vi "Get Result.vi"(8 "error in (no error)":errorcluster, 11 "NI-Scope Lock-in Driver in":refnum<class "NI-Scope Lock-in Driver.lvclass">) -> (0 "error out":errorcluster, 2 "Result":refnum<class "Acquired Result.lvclass">, 3 "NI-Scope Lock-in Driver out":refnum<class "NI-Scope Lock-in Driver.lvclass">)   [LabVIEW 2016, in "NI-Scope Lock-in Driver.lvclass"]
uses:
  NI-Scope Lock-in Driver.lvclass
  C:/github/NHMFL_Core/Libraries/Instruments/Pulse Driver/Pulse Driver.lvclass
  C:/github/NHMFL_Core/Libraries/Instruments/Instrument Driver/Instrument Driver.lvclass
  Instruments/Results/Acquired Result/Acquired Result.lvclass
  Instruments/Results/Start Stream Result/Start Stream Result.lvclass
  C:/github/NHMFL_Core/Libraries/Instruments/Results/Acquired Result/Acquired Result.lvclass
  NI-Scope Lock-in Driver.lvclass/NI-Scope Lock-in Driver.ctl
  Instruments/Pulse Driver/Pulse Driver.lvclass/Pulse Driver.ctl
  Instruments/Instrument Driver/Instrument Driver.lvclass/Instrument Driver.ctl
  Instruments/Results/Start Stream Result/Start Stream Result.lvclass/Start Stream Result.ctl
  Read Sine.vi
  Read Cosine.vi
  Instruments/Pulse Driver/Write Samples per read.vi
  Instruments/Instrument Driver/Read Cycle count.vi
  Instruments/Instrument Driver/Read Cycle period.vi
  Instruments/Results/Start Stream Result/Write Scaling coefficients.vi
  Instruments/Results/Start Stream Result/Write t0.vi
  Instruments/Results/Start Stream Result/Write dt.vi
  Instruments/Results/Start Stream Result/Write Configuration.vi
  Instruments/Instrument Driver/Read User configuration.vi
panel:
  out "Waveform Graph":i16[][](graph)
  out "Current read position":i32
  out "Availiable Samples":u32
  out "Sine waves read":dbl format="%.6g"
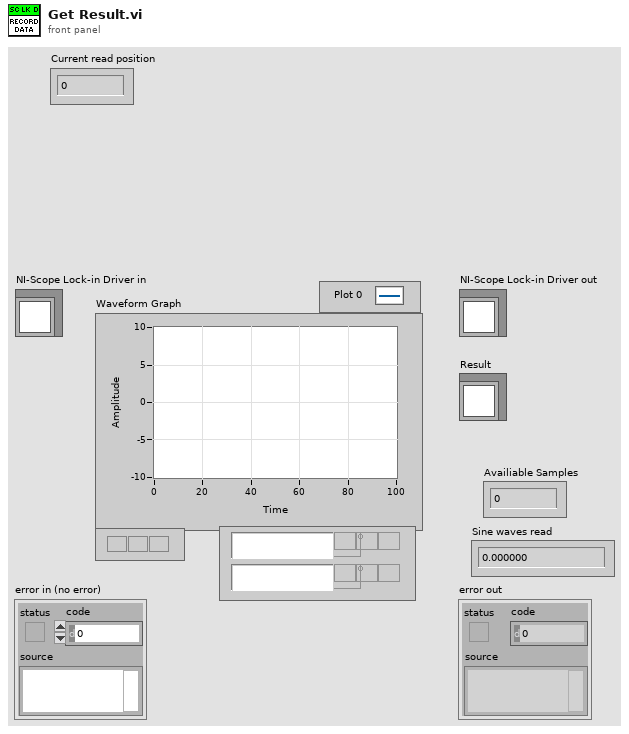
[diagram p1: front panel]
types:
  T1 = typedef "NI-Scope Lock-in Configuration.ctl" = cluster{"Points per sine wave":i32, "Rate":dbl, "Re-name channels":string[], "Active channels":string, "Ranges":dbl[], "Sync on trigger":bool, "R-Q":bool}
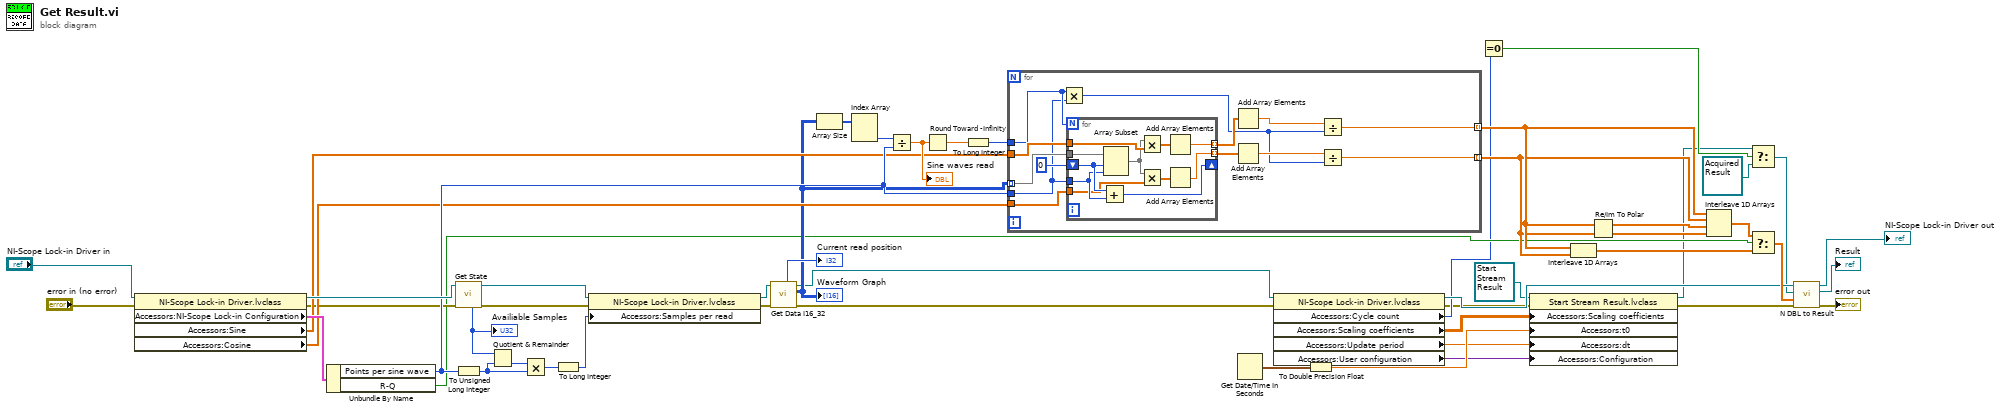
[diagram p0: block diagram]
diagram:
  n1 = property class="NI-Scope Lock-in Driver.lvclass"(reference="NI-Scope Lock-in Driver in", error in="error in (no error)") -> (reference out=w37:refnum<class "NI-Scope Lock-in Driver.lvclass">, error out=w26:errorcluster, "Accessors:NI-Scope Lock-in Configuration"=w36:T1, "Accessors:Sine"=w32:dbl[], "Accessors:Cosine"=w31:dbl[])
  n2 = Unbundle By Name(w36) -> ("Points per sine wave"=w33:i32, "R-Q"=w19:bool)
  n3 = call-dynamic "Get State.vi"("error in (no error)"=w26, "NI-Scope Lock-in Driver in"=w37) -> ("error out"=w46:errorcluster, "NI-Scope Lock-in Driver out"=w48:refnum<class "NI-Scope Lock-in Driver.lvclass">, "Availiable Samples"=w49:u32)  [unwired: 4 in, 3 out]
  "Availiable Samples" <- w49
  n4 = To Unsigned Long Integer(number=w33) -> (unsigned 32bit integer=w43:u32)
  n5 = Quotient & Remainder(x=w49, y=w43) -> (floor(x/y)=w44:u32)  [unwired: 1 out]
  n6 = Multiply(x=w44, y=w43) -> (x*y=w42:u32)
  n7 = To Long Integer(number=w42) -> (32bit integer=w41:i32)
  n8 = property class="NI-Scope Lock-in Driver.lvclass"(reference=w48, error in=w46, "Accessors:Samples per read"=w41) -> (reference out=w47:refnum<class "NI-Scope Lock-in Driver.lvclass">, error out=w45:errorcluster)
  n9 = call-dynamic "Get Data I16_32.vi"("error in (no error)"=w45, "Ni-Scope Digitizer in"=w47) -> ("error out"=w30:errorcluster, "I16 data out"=w24:i16[][], "Ni-Scope Digitizer out"=w15:refnum<class "NI-Scope Lock-in Driver.lvclass">, "Current read position"=→"Current read position":i32)  [unwired: 4 in, 2 out]
  "Waveform Graph" <- w24
  n10 = Array Size(array=w24) -> (size(s)=w40:i32[])
  n11 = Index Array(array=w40) -> (element #2=w39:i32)  [unwired: 2 in, 1 out]
  n12 = Divide(x=w39, y=w33) -> (x/y=w35:dbl)
  "Sine waves read" <- w35
  n13 = Round Toward -Infinity(1:w35) -> (0:w34:dbl)
  n14 = To Long Integer(number=w34) -> (32bit integer=w25:i32)
  n15 = for {
    tunnel: w24 -> [w64] mode=indexing
    tunnel: w33 -> [w57]
    tunnel: w32 -> [w62]
    tunnel: [w56] -> w23 mode=indexing
    tunnel: w31 -> [w59]
    tunnel: [w52] -> w22 mode=indexing
    tunnel: w25 -> [w58]
    n16 = Multiply(x=w58, y=w57) -> (x*y=w53:i32)
    n17 = for {
      N: w58 -> [_]
      tunnel: w64 -> [w75]
      shift-right: [w70] -> _
      shift-left: 0 -> [w72]
      tunnel: w57 -> [w71]
      tunnel: w62 -> [w74]
      tunnel: [w69] -> w61 mode=indexing
      tunnel: [w68] -> w60 mode=indexing
      tunnel: w59 -> [w65]
      n18 = Add(x=w72, y=w71) -> (x+y=w70:i32)
      n19 = Array Subset(array=w75, index=w72, length=w71) -> (w66:i16[])
      n20 = Multiply(x=w66, y=w74) -> (x*y=w73:dbl[])
      n21 = Multiply(x=w66, y=w65) -> (x*y=w67:dbl[])
      n22 = Add Array Elements(numeric array=w73) -> (sum=w69:dbl)
      n23 = Add Array Elements(numeric array=w67) -> (sum=w68:dbl)
    }
    n24 = Add Array Elements(numeric array=w61) -> (sum=w55:dbl)
    n25 = Add Array Elements(numeric array=w60) -> (sum=w54:dbl)
    n26 = Divide(x=w55, y=w53) -> (x/y=w56:dbl)
    n27 = Divide(x=w54, y=w53) -> (x/y=w52:dbl)
  }
  n28 = Get Date/Time In Seconds() -> (seconds since 1Jan1904=w4:timestamp)
  n29 = property class="NI-Scope Lock-in Driver.lvclass"(reference=w15, error in=w30) -> (reference out=w14:refnum<class "NI-Scope Lock-in Driver.lvclass">, error out=w9:errorcluster, "Accessors:Cycle count"=w13:i32, "Accessors:Scaling coefficients"=w10:dbl[][], "Accessors:Update period"=w2:dbl, "Accessors:User configuration"=w1:variant)
  n30 = To Double Precision Float(number=w4) -> (double precision float=w3:dbl)
  n31 = Equal To 0?(x=w13) -> (x = 0?=w12:bool)
  n32 = property class="Start Stream Result.lvclass"(reference=refnum<class "Start Stream Result.lvclass"> refnum ("Start Stream Result.lvclass"), error in=w9, "Accessors:Scaling coefficients"=w10, "Accessors:t0"=w3, "Accessors:dt"=w2, "Accessors:Configuration"=w1) -> (reference out=w7:refnum<class "Start Stream Result.lvclass">, error out=w8:errorcluster)
  n33 = Interleave 1D Arrays(w23, w22) -> (w17:dbl[])
  n34 = Re/Im To Polar(2:w22, 3:w23) -> (0:w20:dbl[], 1:w21:dbl[])
  n35 = Interleave 1D Arrays(w23, w22, w21, w20) -> (w18:dbl[])
  n36 = Select(t=w7, s=w12, f=refnum<class "Acquired Result.lvclass"> refnum ("Acquired Result.lvclass")) -> (s? t:f=w6:refnum<class "Acquired Result.lvclass">)
  n37 = Select(t=w18, s=w19, f=w17) -> (s? t:f=w16:dbl[])
  n38 = call-dynamic "N DBL to Result.vi"("error in (no error)"=w8, "Data"=w16, "Result in"=w6, "Instrument Driver in"=w14) -> ("error out"=→"error out":errorcluster, "Result out"=→"Result":refnum<class "Acquired Result.lvclass">, "Instrument Driver out"=→"NI-Scope Lock-in Driver out":refnum<class "NI-Scope Lock-in Driver.lvclass">)  [unwired: 5 in]
